vi "test_libssh2_session_banner_get.vi"() -> ()   [LabVIEW 2013, in "libssh2_integration_tests.lvlib"]
uses:
  libssh2_integration_tests.lvlib
  <vilib>/addons/_JKI Toolkits/Caraya/classes/Test/Test.lvclass
  libssh2/libssh2.lvlib
  Assert Extensions/Assert Extensions.lvclass
panel:
  out "error out":errorcluster
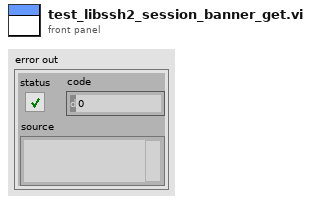
[diagram p1: front panel]
types:
  T1 = typedef "libssh2.lvlib/Session Refnum.ctl" = refnum<k1>
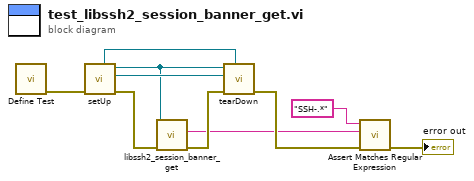
[diagram p0: block diagram]
diagram:
  n1 = call <vilib>:"Define Test.vi"() -> ("error out"=w9:errorcluster)  [unwired: 10 in, 1 out]
  n2 = call "setUp.vi"("error in (no error)"=w9) -> ("error out"=w4:errorcluster, "connection ID"=w8:refnum<k5>, "session"=w6:T1, "fixture"=w7:refnum<class "Server Fixture.lvclass">)  [unwired: 7 in]
  n3 = call "libssh2_session_banner_get.vi"("error in (no error)"=w4, "session"=w6) -> ("error out"=w5:errorcluster, "banner"=w1:string)  [unwired: 8 in]
  n4 = call "tearDown.vi"("fixture"=w7, "error in (no error)"=w5, "connection ID"=w8, "session"=w6) -> ("error out"=w3:errorcluster)  [unwired: 7 in]
  n5 = call "Assert Matches Regular Expression.vi"("error in (no error)"=w3, "Actual Value"=w1, "Regular Expression"="SSH-.*") -> ("error out"=→"error out":errorcluster)  [unwired: 8 in]
